vi "HostDataIndicators (1).vi"(11 "Array":dbl[](array[numeric])) -> (3 "Health Check":T1(array[cluster]))   [LabVIEW 2017]
uses:
  HostDataGLOBAL.vi
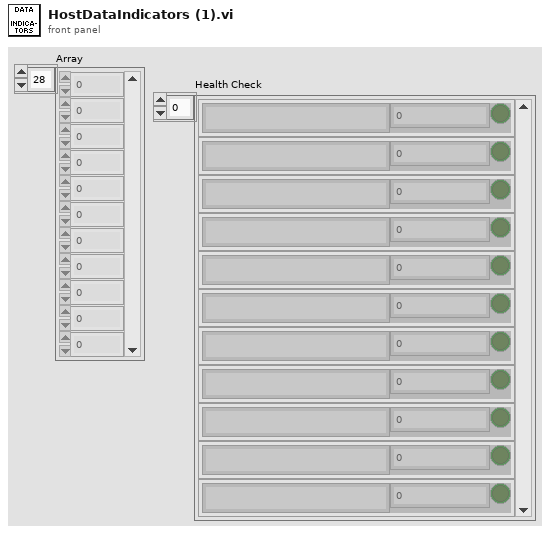
[diagram p1: front panel]
types:
  T1 = cluster{"String":string, "Numeric":dbl, "Boolean":bool}[]
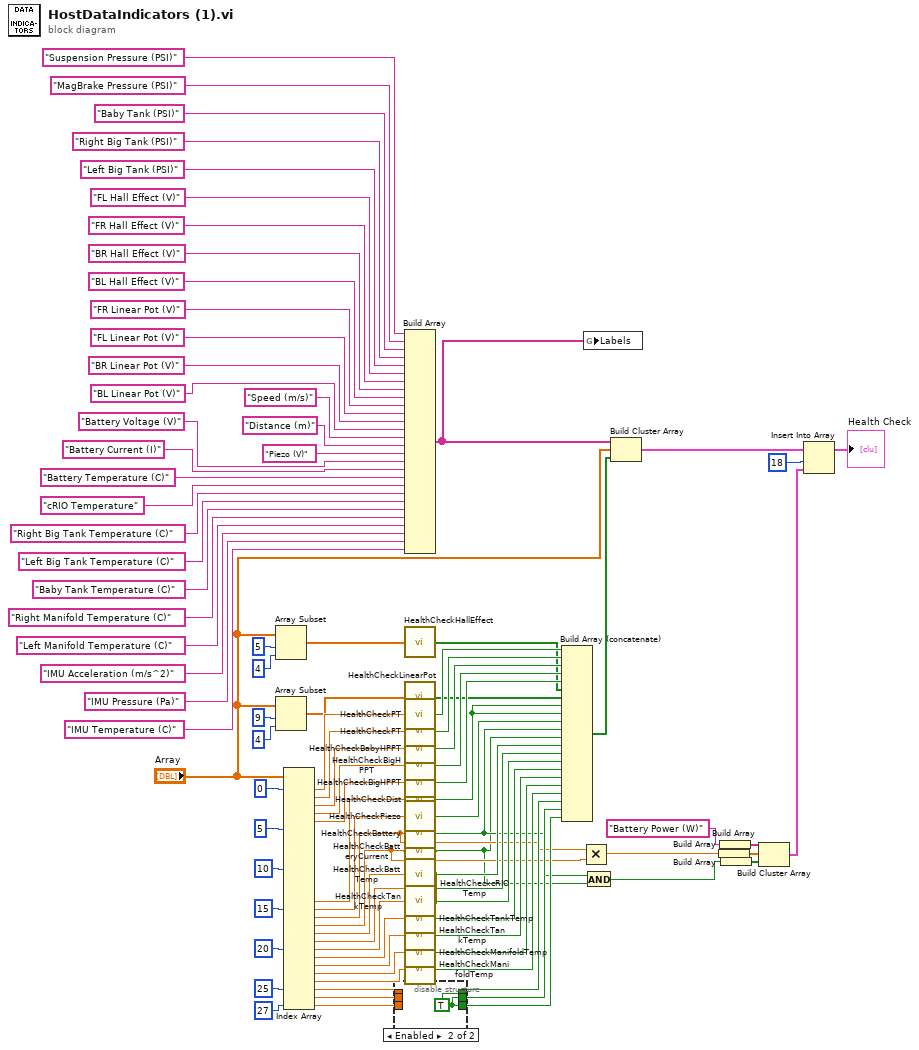
[diagram p0: block diagram]
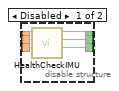
[diagram p2: hidden frame]
diagram:
  n1 = Array Subset(array="Array", index=5, length=4) -> (w48:dbl[])
  n2 = Array Subset(array="Array", index=9, length=4) -> (w45:dbl[])
  n3 = Index Array(array="Array", index #1=0 ("index"), index #6=5 ("index"), index #11=10 ("index"), index #16=15 ("index"), index #21=20 ("index"), index #26=25 ("index"), index #28=27 ("index")) -> (element #1=w62:dbl, element #2=w60:dbl, element #3=w56:dbl, element #4=w54:dbl, element #5=w52:dbl, element #15=w29:dbl, element #16=w32:dbl, element #17=w14:dbl, element #18=w15:dbl, element #19=w17:dbl, element #20=w19:dbl, element #21=w28:dbl, element #22=w27:dbl, element #23=w26:dbl, element #24=w25:dbl, element #25=w24:dbl, element #26=w23:dbl, element #27=w22:dbl, element #28=w21:dbl)  [unwired: 21 in, 9 out]
  n4 = disable-structure shown="Enabled" {
    disable-tunnel: [w100 w101] -> w37
    disable-tunnel: [w99 w101] -> w36
    disable-tunnel: [w98 w101] -> w35
    disable-tunnel: w23 -> [w97 _]
    disable-tunnel: w22 -> [w96 _]
    disable-tunnel: w21 -> [w95 _]
    frame Disabled {
      n5 = call "HealthCheckIMU.vi"("Numeric 3"=w95, "Numeric 2"=w96, "Numeric"=w97) -> ("Boolean 3"=w98:bool, "Boolean 2"=w99:bool, "Boolean"=w100:bool)  [unwired: 6 in]
    }
    frame Enabled {
      w101 = TRUE ("Boolean 3")
    }
  }
  n6 = Build Array("Suspension Pressure (PSI)", "MagBrake Pressure (PSI)", "Baby Tank (PSI)", "Right Big Tank (PSI)", "Left Big Tank (PSI)", "FL Hall Effect (V)", "FR Hall Effect (V)", "BR Hall Effect (V)", "BL Hall Effect (V)", "FR Linear Pot (V)", "FL Linear Pot (V)", "BR Linear Pot (V)", "BL Linear Pot (V)", "Speed (m/s)", "Distance (m)", "Piezo (V)", "Battery Voltage (V)", "Battery Current (I)", "Battery Temperature (C)", "cRIO Temperature", "Right Big Tank Temperature (C)", "Left Big Tank Temperature (C)", "Baby Tank Temperature (C)", "Right Manifold Temperature (C)", "Left Manifold Temperature (C)", "IMU Acceleration (m/s^2)", "IMU Pressure (Pa)", "IMU Temperature (C)") -> (w13:string[])
  n7 = call "HealthCheckHallEffect.vi"("Array"=w48) -> ("Array 2"=w47:bool[])
  n8 = call "HealthCheckLinearPot.vi"("Array"=w45) -> ("Array 2"=w44:bool[])
  n9 = call "HealthCheckPT.vi"("Numeric"=w62) -> ("Boolean"=w61:bool)
  n10 = call "HealthCheckPT.vi"("Numeric"=w60) -> ("Boolean"=w59:bool)
  n11 = call "HealthCheckBabyHPPT.vi"("Numeric"=w56) -> ("Boolean"=w55:bool)
  n12 = call "HealthCheckBigHPPT.vi"("Numeric"=w54) -> ("Boolean"=w53:bool)
  n13 = call "HealthCheckBigHPPT.vi"("Numeric"=w52) -> ("Boolean"=w51:bool)
  n14 = call "HealthCheckDist.vi"("Numeric"=w29) -> ("Boolean"=w31:bool)
  n15 = call "HealthCheckPiezo.vi"("Numeric"=w32) -> ("Boolean"=w30:bool)
  n16 = call "HealthCheckBattery.vi"("Numeric"=w14) -> ("Boolean"=w12:bool)
  n17 = call "HealthCheckBatteryCurrent.vi"("Numeric"=w15) -> ("Boolean"=w11:bool)
  n18 = call "HealthCheckBattTemp.vi"("Numeric"=w17) -> ("Boolean"=w16:bool)
  n19 = call "HealthCheckTankTemp.vi"("Numeric"=w28) -> ("Boolean"=w43:bool)
  n20 = call "HealthCheckTankTemp.vi"("Numeric"=w27) -> ("Boolean"=w42:bool)
  n21 = call "HealthCheckTankTemp.vi"("Numeric"=w26) -> ("Boolean"=w41:bool)
  n22 = call "HealthCheckManifoldTemp.vi"("Numeric"=w25) -> ("Boolean"=w40:bool)
  n23 = call "HealthCheckManifoldTemp.vi"("Numeric"=w24) -> ("Boolean"=w39:bool)
  n24 = call "HealthCheckcRIOTemp.vi"("Numeric"=w19) -> ("Boolean"=w18:bool)
  n25 = Build Array (concatenate)(w61, w59, w55, w53, w51, w47, w44, w31, w31, w30, w12, w11, w16, w18, w43, w42, w41, w40, w39, w37, w36, w35) -> (w68:bool[])
  n26 = Multiply(x=w14, y=w15) -> (x*y=w7:dbl)
  n27 = global write "HostDataGLOBAL.vi" "Labels"(w13) -> ()
  n28 = And(x=w12, y=w11) -> (x .and. y?=w8:bool)
  n29 = Build Cluster Array(w13, "Array", w68) -> (w4:cluster{string, dbl, "Boolean 3":bool}[])
  n30 = Build Array(w7) -> (w6:dbl[])
  n31 = Build Array("Battery Power (W)") -> (w9:string[])
  n32 = Build Array(w8) -> (w5:bool[])
  n33 = Build Cluster Array(w9, w6, w5) -> (w1:cluster{string, dbl, bool}[])
  n34 = Insert Into Array(array=w4, index=18, new element=w1) -> (→"Health Check":cluster{string, dbl, "Boolean 3":bool}[])
